vi "ke37xx Configure Thermocouple.vi"(0 "VISA Resource Name":refnum<visa-resource-name>, 5 "Thermocouple Type (1: K-Type)":T1(ring)=enum."K-Type", 7 "Reference Junction Type (1: Internal)":enum16{"Simulated", "Internal", "External"}(ring)=enum."Internal", 9 "Simulated Reference Temperature (23 degC)":dbl=23.0, 11 "error in (no error)":errorcluster, 12 "Open Detector Enabled (F)":bool) -> (4 "VISA Resource Name Out":refnum<visa-resource-name>, 15 "error out":errorcluster)   [LabVIEW 2009, in "Keithley 3700 Series.lvlib"]
doc: "This VI allows you to configure various aspects of the thermocouple used for temperature measurement."
uses:
  <instrlib>/Keithley 3706/Keithley 3700 Series.lvlib
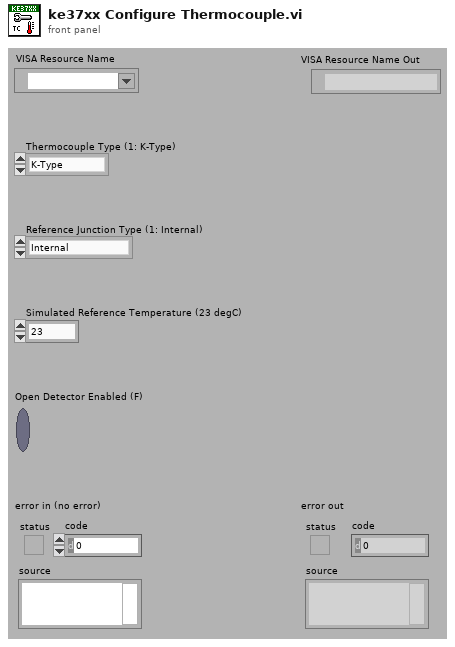
[diagram p1: front panel]
types:
  T1 = enum16{"J-Type", "K-Type", "T-Type", "E-Type", "R-Type", "S-Type", "B-Type", "N-Type"}
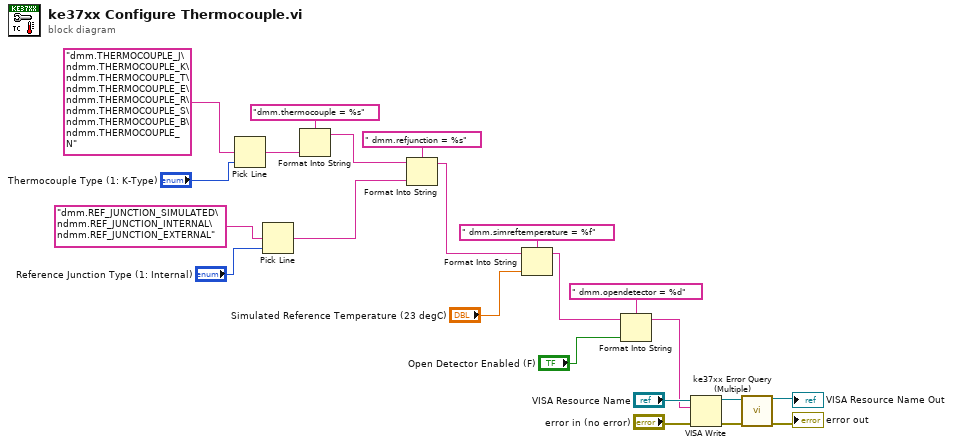
[diagram p0: block diagram]
diagram:
  n1 = Pick Line(multi-line string="dmm.THERMOCOUPLE_J\ndmm.THERMOCOUPLE_K\ndmm.THERMOCOUPLE_T\ndmm.THERMOCOUPLE_E\ndmm.THERMOCOUPLE_R\ndmm.THERMOCOUPLE_S\ndmm.THERMOCOUPLE_B\ndmm.THERMOCOUPLE_N", line index="Thermocouple Type (1: K-Type)") -> (output string=w15:string)  [unwired: 1 out]
  n2 = Pick Line(multi-line string="dmm.REF_JUNCTION_SIMULATED\ndmm.REF_JUNCTION_INTERNAL\ndmm.REF_JUNCTION_EXTERNAL", line index="Reference Junction Type (1: Internal)") -> (output string=w14:string)  [unwired: 1 out]
  n3 = Format Into String(format string="dmm.thermocouple = %s" ("write buffer"), w15) -> (resulting string=w11:string)  [unwired: 2 in, 1 out]
  n4 = Format Into String(format string=" dmm.refjunction = %s" ("write buffer"), initial string=w11, w14) -> (resulting string=w8:string)  [unwired: 1 in, 1 out]
  n5 = Format Into String(format string=" dmm.simreftemperature = %f" ("write buffer"), initial string=w8, "Simulated Reference Temperature (23 degC)") -> (resulting string=w7:string)  [unwired: 1 in, 1 out]
  n6 = Format Into String(format string=" dmm.opendetector = %d" ("write buffer"), initial string=w7, "Open Detector Enabled (F)") -> (resulting string=w3:string)  [unwired: 1 in, 1 out]
  n7 = VISA Write(VISA resource name="VISA Resource Name", write buffer=w3, error in (no error)="error in (no error)") -> (VISA resource name out=w18:refnum<visa-resource-name>, error out=w17:errorcluster)  [unwired: 1 out]
  n8 = call <instrlib>:"ke37xx Error Query (Multiple).vi"("VISA resource name"=w18, "error in (no error)"=w17) -> ("VISA resource name out"=→"VISA Resource Name Out":refnum<visa-resource-name>, "error out"=→"error out":errorcluster)  [unwired: 12 out]
